vi "delate全局.vi"() -> ()   [LabVIEW 2018]
panel:
  in  "startprogram":i32[](array[numeric])
  in  "布尔":bool
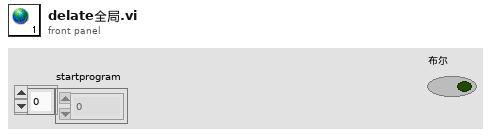
[diagram p1: front panel]
diagram:
